vi "SavePlotData.vi"(8 "error in (no error)":errorcluster caption="错误输入（无错误）", 10 "数据输入":cluster{"数组":dbl[]}[](array[cluster]), 11 "TrendPlot 输入":refnum<class "TrendPlot.lvclass">) -> (0 "error out":errorcluster caption="错误输出", 3 "TrendPlot 输出":refnum<class "TrendPlot.lvclass">)   [LabVIEW 2018, in "DataDisplay.lvlib" / "TrendPlot.lvclass"]
uses:
  TrendPlot.lvclass
  TrendPlot.lvclass/TrendPlot.ctl
  SubVI/WriteDataFile.vi
  DataDisplay.lvlib
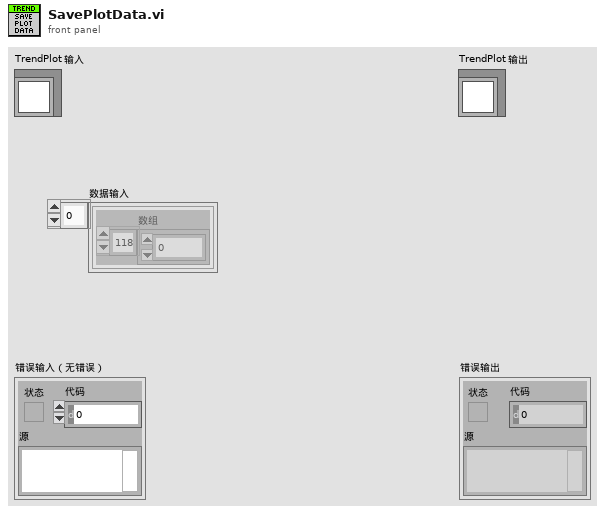
[diagram p1: front panel]
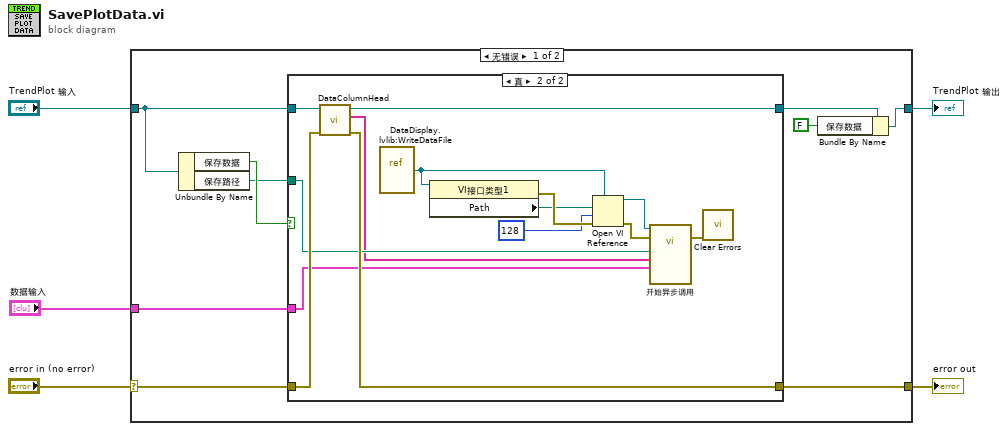
[diagram p0: block diagram]
diagram:
  n1 = case shown="无错误" "error in (no error)" {
    selector: "error in (no error)" -> [w8 w32]
    tunnel: [w7 w32] -> w4
    tunnel: [w9 w31] -> w2
    tunnel: "TrendPlot 输入" -> [w11 w31]
    tunnel: "数据输入" -> [w6 _]
    frame No Error {
      n2 = Unbundle By Name(w11) -> ("保存数据"=w14:bool, "保存路径"=w12:path)
      n3 = case shown="真" w14 {
        tunnel: w12 -> [_ w20]
        tunnel: [w15 w29] -> w10
        tunnel: w11 -> [w15 w30]
        tunnel: [w16 w27] -> w7
        tunnel: w8 -> [w16 w28]
        tunnel: w6 -> [_ w18]
        frame False {
        }
        frame True {
          n4 = call "DataColumnHead.vi"("error in (no error)"=w28, "TrendPlot 输入"=w30) -> ("error out"=w27:errorcluster, "首行"=w19:string[], "TrendPlot 输出"=w29:refnum<class "TrendPlot.lvclass">)  [unwired: 7 in]
          n5 = vi-ref "DataDisplay.lvlib:WriteDataFile.vi"() -> (w25:refnum<vi>)
          n6 = property class="VI接口类型1"(reference=w25) -> (error out=w26:errorcluster, "Path"=w24:path)  [unwired: 1 in, 1 out]
          n7 = Open VI Reference(type specifier VI Refnum (for type only)=w25, vi path=w24, options=128 ("选项"), error in (no error)=w26) -> (vi reference=w22:refnum<vi>, error out=w21:errorcluster)  [unwired: 2 in]
          n8 = call-by-ref "开始异步调用"(reference=w22, error in=w21, "数据输入"=w18, "首行"=w19, "保存路径"=w20) -> (error out=w17:errorcluster)  [unwired: 9 in, 1 out]
          n9 = call <vilib>:"Clear Errors.vi"("error in (no error)"=w17) -> ()  [unwired: 5 in, 2 out]
        }
      }
      n10 = Bundle By Name(cluster=w10, "保存数据"=FALSE) -> (w9:refnum<class "TrendPlot.lvclass">)
    }
    frame Error {
    }
  }
  "error out" <- w4
  "TrendPlot 输出" <- w2
